vi "Increment.vi"(6 "Labels":map{string, string}(c390), 8 "error in (no error)":errorcluster, 10 "Step":dbl=1.0, 11 "Counter Ref":refnum<data-value>) -> (0 "error out":errorcluster, 3 "Counter Ref out":refnum<data-value>)   [LabVIEW 2020, in "Metrics.lvlib" / "Counter.lvclass"]
doc: "Increments the value of the counter. By default, the increment value is 1."
uses:
  Counter.lvclass
  C:/Github-locals/PromVIEW/src/metrics/metric/Metric.lvclass
  sample/Edit Action.ctl
  metric/Metric.lvclass
  sample/Sample.lvclass
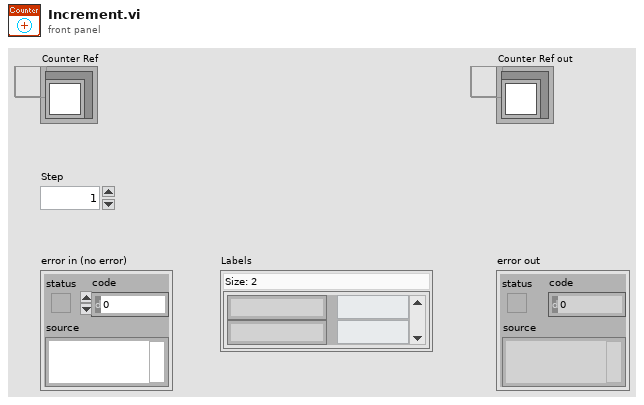
[diagram p1: front panel]
types:
  T1 = typedef "Metrics.lvlib/Sample.lvclass/Edit Action.ctl" = enum16{"Set", "Increment"}
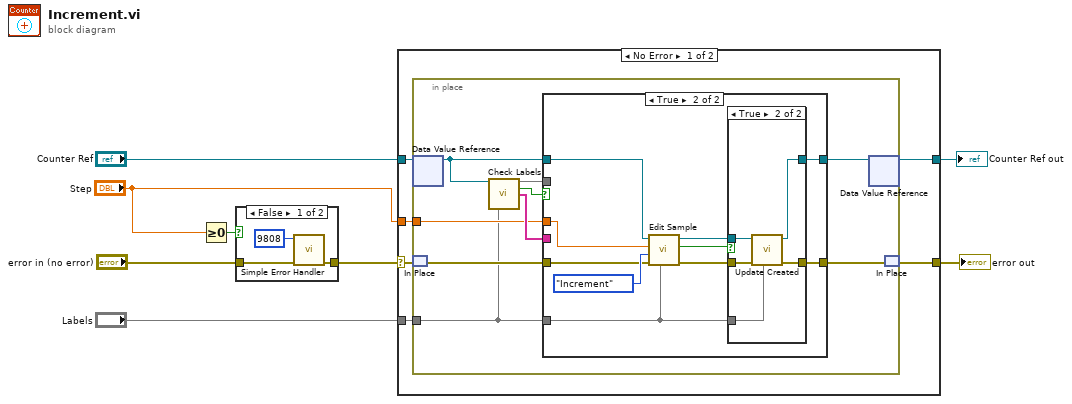
[diagram p0: block diagram]
diagram:
  n1 = Greater Or Equal To 0?(x="Step") -> (x >= 0?=w7:bool)
  n2 = case shown="False" w7 {
    tunnel: "error in (no error)" -> [w10 w12]
    tunnel: [w9 w12] -> w5
    frame False {
      n3 = call <vilib>:"Simple Error Handler.vi"("error code (no error:0)"=9808, "error in (no error)"=w10) -> ("error out"=w9:errorcluster)  [unwired: 3 in, 4 out]
    }
    frame True {
    }
  }
  n4 = case shown="No Error" w5 {
    selector: w5 -> [w17 w47]
    tunnel: "Counter Ref" -> [w18 w48]
    tunnel: "Labels" -> [w16 _]
    tunnel: "Step" -> [w15 _]
    tunnel: [w14 w47] -> w2
    tunnel: [w13 w48] -> w1
    frame No Error {
      n5 = in-place {
        in-place-border: w16 -> [w21]
        in-place-border: w15 -> [w22]
        n6 = in-place-dvr #1(w18) -> (w27:refnum<class "Counter.lvclass">)  [unwired: 1 out]
        n7 = in-place-match #2(w17) -> (w26:errorcluster)
        n8 = call-dynamic "Check Labels.vi"("Metric in"=w27, "Labels"=w21) -> ("Samples"=w23:map{string, refnum<class "Sample.lvclass">}, "Valid Labels"=w24:bool, "Label Values"=w25:string[])  [unwired: 11 in]
        n9 = case shown="True" w24 {
          tunnel: w25 -> [_ _]
          tunnel: w23 -> [_ _]
          tunnel: w22 -> [_ w36]
          tunnel: w21 -> [_ w30]
          tunnel: w26 -> [w29 w34]
          tunnel: [w29 w39] -> w20
          tunnel: w27 -> [w28 w37]
          tunnel: [w28 w38] -> w19
          frame False {
          }
          frame True {
            n10 = call "Edit Sample.vi"("Labels"=w30, "error in (no error)"=w34, "Action"=Edit_Action."Increment", "Step"=w36, "Metric in"=w37) -> ("error out"=w31:errorcluster, "New Sample?"=w32:bool, "Metric out"=w33:refnum<class "Counter.lvclass">)  [unwired: 4 in]
            n11 = case shown="True" w32 {
              tunnel: w31 -> [w41 w46]
              tunnel: [w41 w45] -> w39
              tunnel: w30 -> [_ w44]
              tunnel: w33 -> [w40 w43]
              tunnel: [w40 w42] -> w38
              frame False {
              }
              frame True {
                n12 = call "Update Created.vi"("Labels"=w44, "error in (no error)"=w46, "Counter in"=w43) -> ("error out"=w45:errorcluster, "Counter out"=w42:refnum<class "Counter.lvclass">)  [unwired: 7 in]
              }
            }
          }
        }
        n13 = in-place-dvr #1(w19) -> (w13:refnum<data-value>)  [unwired: 1 out]
        n14 = in-place-match #2(w20) -> (w14:errorcluster)
      }
    }
    frame Error {
    }
  }
  "error out" <- w2
  "Counter Ref out" <- w1
